vi "Lift Test.vi"(10 "Run?":bool) -> ()   [LabVIEW 2018]
uses:
  SubSystems/Lift/Lift Global.vi
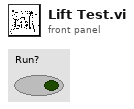
[diagram p1: front panel]
types:
  T1 = enum16{"Manual", "Hatch Panel Zone 1", "Hatch Panel Zone 2", "Hatch Panel Zone 3", "Cargo Zone 1", "Cargo Zone 2", "Cargo Zone 3", "Cargo Ship Zone"}
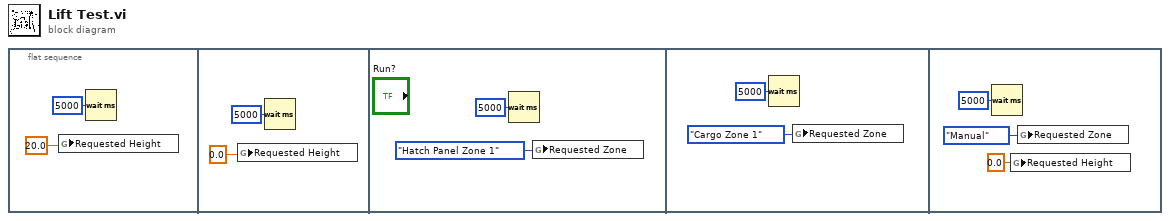
[diagram p0: block diagram]
diagram:
  n1 = flat-sequence {
    frame #0 {
      n2 = global write "Lift Global.vi" "Requested Height"(20.0 ("Requested Height")) -> ()
      n3 = Wait (ms)(milliseconds to wait=u32 5000) -> ()  [unwired: 1 out]
    }
    frame #1 {
      n4 = global write "Lift Global.vi" "Requested Height"(0.0 ("Requested Height")) -> ()
      n5 = Wait (ms)(milliseconds to wait=u32 5000) -> ()  [unwired: 1 out]
    }
    frame #2 {
      n6 = Wait (ms)(milliseconds to wait=u32 5000) -> ()  [unwired: 1 out]
      n7 = global write "Lift Global.vi" "Requested Zone"(T1."Hatch Panel Zone 1" ("Requested Zone")) -> ()
    }
    frame #3 {
      n8 = Wait (ms)(milliseconds to wait=u32 5000) -> ()  [unwired: 1 out]
      n9 = global write "Lift Global.vi" "Requested Zone"(T1."Cargo Zone 1" ("Requested Zone")) -> ()
    }
    frame #4 {
      n10 = Wait (ms)(milliseconds to wait=u32 5000) -> ()  [unwired: 1 out]
      n11 = global write "Lift Global.vi" "Requested Height"(0.0 ("Requested Height")) -> ()
      n12 = global write "Lift Global.vi" "Requested Zone"(T1."Manual" ("Requested Zone")) -> ()
    }
  }
